vi "OnUpdateMenu.vi"(8 "error in (no error)":errorcluster, 11 "Game in":refnum<class "Game.lvclass">) -> (0 "error out":errorcluster, 3 "Game out":refnum<class "Game.lvclass">)   [LabVIEW 2019, in "RT_Game.lvlib" / "Game.lvclass"]
uses:
  Game.lvclass
  Game.lvclass/Game.ctl
  GameMenu/GameMenu.lvclass
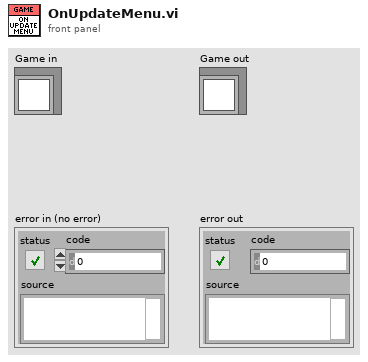
[diagram p1: front panel]
types:
  T1 = typedef "RT_Game.lvlib/Game.lvclass/States.ctl" = enum16{"Init", "Restart", "Menu", "Game", "Resume", "ToggleSingleplayer", "LoadNextGame", "ExitToMenu", "NewHighscore", "GameOver", "SlideOut"}
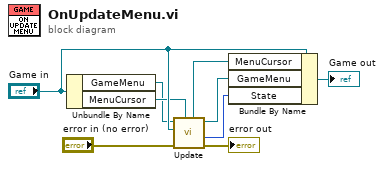
[diagram p0: block diagram]
diagram:
  n1 = Unbundle By Name("Game in") -> ("GameMenu"=w2:refnum<class "GameMenu.lvclass">, "MenuCursor"=w6:refnum<class "RT_Sprite.lvclass">)
  n2 = call-dynamic "Update.vi"("CursorIn"=w6, "error in (no error)"="error in (no error)", "Game(readonly)"="Game in", "GameMenu in"=w2) -> ("error out"=→"error out":errorcluster, "State"=w5:T1, "GameMenu out"=w3:refnum<class "GameMenu.lvclass">, "CursorOut"=w7:refnum<class "RT_Sprite.lvclass">)  [unwired: 4 in]
  n3 = Bundle By Name(cluster="Game in", "MenuCursor"=w7, "GameMenu"=w3, "State"=w5) -> (→"Game out":refnum<class "Game.lvclass">)
